vi "Gr_resistance_lockin_using_Rbox_probe.vi"() -> ()   [LabVIEW 2024]
uses:
  <vilib>/Analysis/1siggen.llb/Ramp Pattern by Delta.vi
  <vilib>/Utility/file.llb/Write Delimited Spreadsheet (DBL).vi
  <vilib>/Utility/file.llb/Write Delimited Spreadsheet (string).vi
  <vilib>/Analysis/NI_AALBase.lvlib
  <vilib>/Analysis/NI_AALPro.lvlib
  C:/Users/Public/OneDrive/Desktop/Keithley_2450_2470_1_4_0_LV2015_NewReadme2_2450-LV2015-1.4.0/Keithley 2450/Keithley 2450.lvlib
panel:
  out "Rgr vs Vb":cluster{dbl[], dbl[]}(graph)
  in  "Measurement Count":u32=10
  in  "reset?":bool
  in  "save data":string="H:\\My Drive\\Lab\\PPMS\\Measurement\\GaN_1000C_2min_34_56"
  in  "lockin_avgs":i32=10
  out "std voltage measured":dbl format="%0.2f"
  out "mean voltage measured":dbl=6.7979141 format="%0.4f"
  out "std current measured":dbl=1.0038305493714546e-08 format="%0.5e"
  out "mean current measured":dbl=1.7421272433999997e-09 format="%.4e"
  in  "VISA resource name 2450":refnum<visa-resource-name>="GPIB0::1::INSTR"
  in  "Current Limit":dbl=5e-08
  out "Vb":dbl
  in  "loop?":bool=TRUE
  in  "Vb end (V)":dbl format="%#.4f"
  in  "Vb step (mV)":dbl format="%#_4f"
  in  "Vb start (V)":dbl format="%#.4f"
  out "R_gr":dbl
  out "slope":dbl format="%#_14f"
  out "Vdev":dbl format="%#_14f"
  in  "lockinwait":u32=50
  out "Vbox":dbl format="%#_14f"
  out "Vref vs Idev":cluster{dbl[], dbl[]}[](graph)
  out "Ibox":dbl format="%#_14f"
  in  "Rbox":dbl format="%#_20f"
  out "Sin voltage in":dbl=1.0 format="%#_13f"
  in  "Vmax":dbl format="%.3f"
  in  "Vstep":dbl format="%.5f"
  in  "Vmin":dbl format="%.3f"
  in  "A frequency":dbl=26.7 format="%#_13g"
  in  "B input Connection":u16(ring)=1 items=["Single-Ended Voltage", "Differential Voltage", "1 MOhm Current Gain", "100 MOhm Current Gain"]
  in  "B Reference Source":u8(ring)=1 items=["External", "Internal", "Internal Sweep"]
  in  "B Sensitivity":u16(ring)=26 items=["1 nV/fA", "2 nV/fA", "5 nV/fA", "10 nV/fA", "20 nV/fA", "50 nV/fA", "100 nV/fA", "200 nV/fA", "500 nV/fA", "1 uV/pA", "2 uV/pA", "5 uV/pA", "10 uV/pA", "20 uV/pA", "50 uV/pA", "100 uV/pA", "200 uV/pA", "500 uV/pA", "1 mV/nA", "2 mV/nA", "5 mV/nA", "10 mV/nA", "20 mV/nA", "50 mV/nA", "100 mV/nA", "200 mV/nA", "500 mV/nA", "1 V/uA"]
  in  "LOCKIN1 address":refnum<visa-resource-name>="COM3"
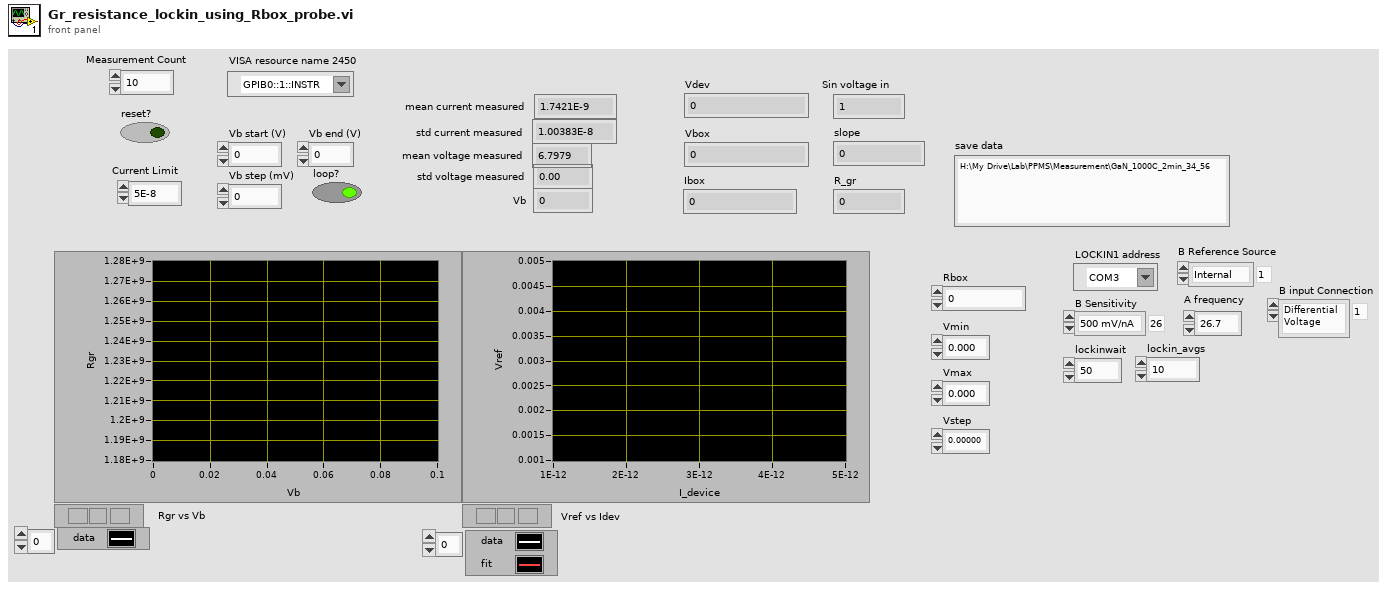
[diagram p1: front panel]
types:
  T1 = enum16{"open", "replace", "create", "open or create", "replace or create", "replace or create with confirmation"}
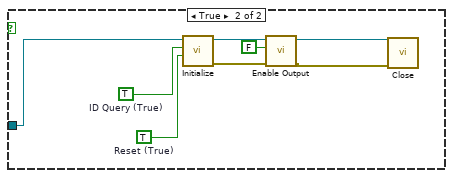
[diagram p3: hidden frame]
diagram:
  w2 = 0
  n1 = Initialize Array(w2, w2) -> (w1:i32[])
  n2 = case shown="False" "reset?" {
    tunnel: "VISA resource name 2450" -> [w10 w581]
    tunnel: w1 -> [w9 _]
    frame False {
      w7 = 0
      w8 = 0
      w17 = TRUE
      n3 = Negate(x="Vb step (mV)") -> (-x=w28:dbl)
      n4 = call-poly <vilib>:"Ramp Pattern.vi"("start"="Vb start (V)", "end"="Vb end (V)", "delta"="Vb step (mV)") -> ("samples"=w24:i32, "Ramp Pattern"=w26:dbl[])  [unwired: 6 in, 1 out]
      n5 = call-poly <vilib>:"Ramp Pattern.vi"("start"="Vb end (V)", "end"="Vb start (V)", "delta"=w28) -> ("samples"=w23:i32, "Ramp Pattern"=w25:dbl[])  [unwired: 6 in, 1 out]
      n6 = case shown="True" "loop?" {
        tunnel: w26 -> [w31 w38]
        tunnel: w25 -> [_ w37]
        tunnel: [w31 w33] -> w20
        tunnel: w24 -> [w32 w35]
        tunnel: [w32 w34] -> w21
        tunnel: w23 -> [_ w36]
        frame False {
        }
        frame True {
          n7 = Add(x=w35, y=w36) -> (x+y=w34:i32)
          n8 = Build Array (concatenate)(w38, w37) -> (w33:dbl[])
        }
      }
      n9 = Concatenate Strings("save data", ".txt" ("string")) -> (w12:string)
      n10 = String To Path(string=w12) -> (path=w19:path)
      n11 = call-poly <vilib>:"Write Delimited Spreadsheet.vi"("file path (dialog if empty)"=w19, "append to file? (new file:F)"=w17) -> ("new file path (Not A Path if cancelled)"=w18:path)  [unwired: 12 in, 1 out]
      n12 = Build Array("# Vb_set(V) Vb_meas(V) R_Gr(Ohm) Ib(uA) " ("string")) -> (w15:string[])
      n13 = Initialize Array(w7, w7) -> (w6:i32[])
      n14 = Initialize Array(w8, w8) -> (w5:i32[])
      n15 = call-poly <vilib>:"Write Delimited Spreadsheet.vi"("file path (dialog if empty)"=w18, "1D data"=w15, "append to file? (new file:F)"=w17) -> ("new file path (Not A Path if cancelled)"=w14:path)  [unwired: 11 in, 1 out]
      n16 = for {
        N: w21 -> [_]
        tunnel: w20 -> [w71] mode=indexing
        tunnel: w10 -> [w99]
        tunnel: w14 -> [w98]
        tunnel: "save data" -> [w81]
        shift-right: [w62] -> _
        shift-left: w9 -> [w72]
        shift-right: [w40] -> _
        shift-left: w6 -> [w59]
        shift-right: [w43] -> _
        shift-left: w5 -> [w52]
        i -> [w39]
        n17 = flat-sequence {
          tunnel: w71 -> [w142]
          tunnel: [w142] -> w100
          tunnel: w99 -> [w154]
          tunnel: [w153] -> w88
          tunnel: [w152] -> w82
          tunnel: w72 -> [w143]
          tunnel: w71 -> [_]
          tunnel: [w143] -> w68
          tunnel: [w140] -> w60
          tunnel: w59 -> [w139]
          tunnel: [w139] -> w58
          tunnel: w52 -> [w138]
          tunnel: [w138] -> w46
          tunnel: [w262] -> w131
          tunnel: [w261] -> w130
          tunnel: ["Rbox"] -> w102
          tunnel: [w257] -> w129
          tunnel: ["Rbox"] -> w128
          tunnel: [w248] -> w127
          tunnel: w100 -> [w248]
          tunnel: [w254] -> w89
          tunnel: w88 -> [w254]
          tunnel: [w253] -> w83
          tunnel: w82 -> [w253]
          tunnel: w81 -> [w252]
          tunnel: ["A frequency"] -> w79
          tunnel: [w250] -> w73
          tunnel: [w249] -> w69
          tunnel: w68 -> [w249]
          tunnel: w60 -> [_]
          tunnel: w58 -> [w244]
          tunnel: [w244] -> w57
          tunnel: [w243] -> w47
          tunnel: w46 -> [w243]
          tunnel: w39 -> [w240]
          tunnel: w131 -> [w296]
          tunnel: [w296] -> w126
          tunnel: w130 -> [w295]
          tunnel: [w295] -> w125
          tunnel: [w279] -> w124
          tunnel: w129 -> [w294]
          tunnel: w128 -> [w291]
          tunnel: ["lockinwait"] -> w101
          tunnel: w127 -> [w273]
          tunnel: [w273] -> w94
          tunnel: [w272] -> w90
          tunnel: w89 -> [w272]
          tunnel: [w271] -> w84
          tunnel: w83 -> [w271]
          tunnel: [w269] -> w80
          tunnel: w79 -> [w269]
          tunnel: [w267] -> w74
          tunnel: w73 -> [w267]
          tunnel: [w266] -> w70
          tunnel: w69 -> [w266]
          tunnel: w57 -> [w265]
          tunnel: [w265] -> w56
          tunnel: [w264] -> w48
          tunnel: w47 -> [w264]
          tunnel: [w320] -> w123
          tunnel: [w314] -> w122
          tunnel: w126 -> [w312]
          tunnel: w125 -> [w313]
          tunnel: [w311] -> w121
          tunnel: w124 -> [w311]
          tunnel: [w304] -> w95
          tunnel: w94 -> [w304]
          tunnel: [w303] -> w91
          tunnel: w90 -> [w303]
          tunnel: [w302] -> w85
          tunnel: w84 -> [w302]
          tunnel: w80 -> [w301]
          tunnel: [w300] -> w75
          tunnel: w74 -> [w300]
          tunnel: w70 -> [w299]
          tunnel: [w299] -> w66
          tunnel: w56 -> [w298]
          tunnel: [w298] -> w55
          tunnel: [w297] -> w49
          tunnel: w48 -> [w297]
          tunnel: w123 -> [w331]
          tunnel: w122 -> [w332]
          tunnel: [w332] -> w120
          tunnel: [w331] -> w119
          tunnel: [w330] -> w118
          tunnel: w121 -> [w330]
          tunnel: [w328] -> w96
          tunnel: w95 -> [w328]
          tunnel: [w327] -> w92
          tunnel: w91 -> [w327]
          tunnel: [w326] -> w86
          tunnel: w85 -> [w326]
          tunnel: [w325] -> w76
          tunnel: w75 -> [w325]
          tunnel: [w324] -> w67
          tunnel: w66 -> [w324]
          tunnel: w55 -> [w323]
          tunnel: [w323] -> w54
          tunnel: [w322] -> w50
          tunnel: w49 -> [w322]
          tunnel: w104 -> [w357]
          tunnel: w103 -> [w356]
          tunnel: w120 -> [w355]
          tunnel: w119 -> [w354]
          tunnel: w118 -> [w353]
          tunnel: [w346] -> w117
          tunnel: [w345] -> w116
          tunnel: [w344] -> w115
          tunnel: [w343] -> w114
          tunnel: [w343] -> w113
          tunnel: [w342] -> w112
          tunnel: w102 -> [w341]
          tunnel: w101 -> [w340]
          tunnel: [w339] -> w97
          tunnel: w96 -> [w339]
          tunnel: [w338] -> w93
          tunnel: w92 -> [w338]
          tunnel: [w337] -> w87
          tunnel: w86 -> [w337]
          tunnel: [w336] -> w77
          tunnel: w76 -> [w336]
          tunnel: w67 -> [w335]
          tunnel: [w335] -> w64
          tunnel: w54 -> [w334]
          tunnel: [w334] -> w53
          tunnel: [w333] -> w51
          tunnel: w50 -> [w333]
          tunnel: w117 -> [w543]
          tunnel: w116 -> [w544]
          tunnel: w115 -> [w549]
          tunnel: w114 -> [w550]
          tunnel: w113 -> [w551]
          tunnel: w112 -> [w555]
          tunnel: [w541] -> w111
          tunnel: [w540] -> w110
          tunnel: w98 -> [w539]
          tunnel: w97 -> [w528]
          tunnel: w93 -> [w538]
          tunnel: w87 -> [w537]
          tunnel: [w534] -> w78
          tunnel: w77 -> [w534]
          tunnel: [w532] -> w65
          tunnel: w64 -> [w532]
          tunnel: [w528] -> w61
          tunnel: w53 -> [w530]
          tunnel: w51 -> [w529]
          tunnel: [w527] -> w44
          tunnel: [w526] -> w41
          tunnel: [w574] -> w109
          tunnel: w111 -> [w574]
          tunnel: [w573] -> w108
          tunnel: w110 -> [w573]
          tunnel: w78 -> [w570]
          tunnel: w65 -> [w564]
          tunnel: [w562] -> w63
          tunnel: w61 -> [w563]
          tunnel: [w560] -> w45
          tunnel: w44 -> [w560]
          tunnel: [w559] -> w42
          tunnel: w41 -> [w559]
          tunnel: w109 -> [w580]
          tunnel: w108 -> [w579]
          tunnel: [w578] -> w62
          tunnel: w63 -> [w578]
          tunnel: [w577] -> w43
          tunnel: w45 -> [w577]
          tunnel: [w576] -> w40
          tunnel: w42 -> [w576]
          frame #0 {
            n18 = flat-sequence {
              tunnel: w154 -> [w170]
              tunnel: w142 -> [w155]
              tunnel: [w164] -> w137
              tunnel: [w163] -> w135
              tunnel: ["Measurement Count"] -> w133
              tunnel: w137 -> [w192]
              tunnel: [w192] -> w136
              tunnel: w135 -> [w191]
              tunnel: [w191] -> w134
              tunnel: w133 -> [w190]
              tunnel: [w190] -> w132
              tunnel: [w194] -> w151
              tunnel: w136 -> [w199]
              tunnel: w134 -> [w198]
              tunnel: [w197] -> w150
              tunnel: [w196] -> w149
              tunnel: w132 -> [w193]
              tunnel: [w193] -> w144
              tunnel: [w214] -> w148
              tunnel: w151 -> [w213]
              tunnel: [w213] -> w147
              tunnel: w150 -> [w219]
              tunnel: w149 -> [w218]
              tunnel: [w217] -> w146
              tunnel: [w216] -> w145
              tunnel: w144 -> [w211]
              tunnel: [w232] -> w153
              tunnel: w148 -> [w232]
              tunnel: [w231] -> w152
              tunnel: w147 -> [w231]
              tunnel: w146 -> [w234]
              tunnel: w145 -> [w235]
              frame #0 {
                w172 = u16 2 items=["Volts", "Current", "Resistance"] ("Function (0: Volts)")
                w179 = u16 0 items=["Voltage", "Current"]  # Source Mode  (0: Voltage)
                w180 = u16 1 items=["Volts", "Current", "Auto Resistance", "Manual Resistance", "Digitize Voltage", "Digitize Current"]  # Measurement Mode
                w171 = TRUE  # Enable Auto Range (T:Enable)
                w181 = u16 1 items=["Volts", "Current", "Resistance"]  # Function (0: Volts)
                w182 = u16 0 items=["Volts", "Current", "Resistance"]  # Function (0: Volts)
                w177 = FALSE  # Reset (True)
                n19 = call "Initialize.vi"("Reset (True)"=w177, "VISA resource name"=w170) -> ("error out"=w156:errorcluster, "VISA resource name out"=w161:refnum<visa-resource-name>)  [unwired: 8 in]
                n20 = call "Clear Buffer.vi"("VISA resource name"=w161, "error in (no error)"=w156) -> ("VISA resource name out"=w160:refnum<visa-resource-name>, "error out"=w157:errorcluster)  [unwired: 12 in]
                n21 = call "Clear Buffer Statistics.vi"("VISA resource name"=w160, "error in (no error)"=w157) -> ("VISA resource name out"=w159:refnum<visa-resource-name>, "error out"=w158:errorcluster)  [unwired: 12 in]
                n22 = call "Configure Measurement Range.vi"("error in (no error)"=w158, "Enable Auto Range (T:Enable)"=w171, "Function (0: Volts)"=w182, "VISA resource name"=w159) -> ("error out"=w184:errorcluster, "VISA resource name out"=w183:refnum<visa-resource-name>)  [unwired: 6 in]
                n23 = call "Configure Measurement Range.vi"("error in (no error)"=w184, "Enable Auto Range (T:Enable)"=w171, "Function (0: Volts)"=w181, "VISA resource name"=w183) -> ("error out"=w175:errorcluster, "VISA resource name out"=w176:refnum<visa-resource-name>)  [unwired: 6 in]
                n24 = call "Configure Measurement Range.vi"("error in (no error)"=w175, "Enable Auto Range (T:Enable)"=w171, "Function (0: Volts)"=w172, "VISA resource name"=w176) -> ("error out"=w174:errorcluster, "VISA resource name out"=w173:refnum<visa-resource-name>)  [unwired: 6 in]
                n25 = call "Configure Output.vi"("VISA resource name"=w173, "Source Level (0)"=w155, "Source Mode  (0: Voltage)"=w179, "Source Limit Level (0.1)"="Current Limit", "error in (no error)"=w174) -> ("VISA resource name out"=w185:refnum<visa-resource-name>, "error out"=w186:errorcluster)  [unwired: 9 in]
                n26 = call "Configure Source Function.vi"("error in (no error)"=w186, "Function (0: Volts)"=w179, "VISA resource name"=w185) -> ("error out"=w187:errorcluster, "VISA resource name out"=w188:refnum<visa-resource-name>)  [unwired: 7 in]
                n27 = call "Configure Measurement Function.vi"("error in (no error)"=w187, "Function (0: Volts)"=w180, "VISA resource name"=w188) -> ("error out"=w168:errorcluster, "VISA resource name out"=w169:refnum<visa-resource-name>)  [unwired: 7 in]
                n28 = call "Set Measurement Count.vi"("error in (no error)"=w168, "Measurement Count"="Measurement Count", "VISA resource name"=w169) -> ("error out"=w166:errorcluster, "VISA resource name out"=w167:refnum<visa-resource-name>)  [unwired: 7 in]
                n29 = call "Enable Output.vi"("error in (no error)"=w166, "Enable Output (T: Enable)"=TRUE, "VISA resource name"=w167) -> ("error out"=w163:errorcluster, "VISA resource name out"=w164:refnum<visa-resource-name>)  [unwired: 7 in]
              }
              frame #1 {
                n30 = Wait (ms)(milliseconds to wait=200) -> ()  [unwired: 1 out]
              }
              frame #2 {
                w200 = 1000000.0 ("Timeout (10000 ms)")
                n31 = call "Make Reading and Store in Buffer.vi"("VISA resource name"=w199, "error in (no error)"=w198) -> ("VISA resource name out"=w208:refnum<visa-resource-name>, "error out"=w209:errorcluster)  [unwired: 12 in]
                n32 = call "Read (Multiple Points).vi"("VISA resource name"=w208, "Start Index (1)"=u32 1, "End Index (1)"=w193, "error in (no error)"=w209) -> ("VISA resource name out"=w197:refnum<visa-resource-name>, "Data out"=w203:string, "error out"=w196:errorcluster)  [unwired: 9 in]
                n33 = Spreadsheet String To Array(delimiter (Tab)=",", format string="%s", spreadsheet string=w203, array type (2D Dbl)=dbl[] []) -> (array=w202:dbl[])
                n34 = call <vilib>:"Std Deviation and Variance.vi"("X"=w202) -> ("mean"=w195:dbl, "standard deviation"=w201:dbl)  [unwired: 1 in, 1 out]
                "mean current measured" <- w195
                "std current measured" <- w201
                n35 = Multiply(x=w201, y=w200) -> ()  [unwired: 1 out]
                n36 = Multiply(x=w200, y=w195) -> (x*y=w194:dbl)
              }
              frame #3 {
                n37 = call "Configure Measurement Function.vi"("error in (no error)"=w218, "VISA resource name"=w219) -> ("error out"=w226:errorcluster, "VISA resource name out"=w230:refnum<visa-resource-name>)  [unwired: 8 in]
                n38 = call "Set Measurement Count.vi"("error in (no error)"=w226, "Measurement Count"=w211, "VISA resource name"=w230) -> ("error out"=w227:errorcluster, "VISA resource name out"=w225:refnum<visa-resource-name>)  [unwired: 7 in]
                n39 = Increment(x=w211) -> (x+1=w212:u32)
                n40 = Add(x=w211, y=w211) -> (x+y=w210:u32)
                n41 = call "Make Reading and Store in Buffer.vi"("VISA resource name"=w225, "error in (no error)"=w227) -> ("VISA resource name out"=w229:refnum<visa-resource-name>, "error out"=w228:errorcluster)  [unwired: 12 in]
                n42 = call "Read (Multiple Points).vi"("VISA resource name"=w229, "Start Index (1)"=w212, "End Index (1)"=w210, "error in (no error)"=w228) -> ("VISA resource name out"=w216:refnum<visa-resource-name>, "Data out"=w221:string, "error out"=w217:errorcluster)  [unwired: 9 in]
                n43 = Spreadsheet String To Array(delimiter (Tab)=",", format string="%s", spreadsheet string=w221, array type (2D Dbl)=dbl[] []) -> (array=w220:dbl[])
                n44 = call <vilib>:"Std Deviation and Variance.vi"("X"=w220) -> ("mean"=w214:dbl, "standard deviation"=→"std voltage measured":dbl)  [unwired: 1 in, 1 out]
                "mean voltage measured" <- w214
              }
              frame #4 {
                n45 = call "Enable Output.vi"("error in (no error)"=w234, "Enable Output (T: Enable)"=TRUE, "VISA resource name"=w235) -> ("error out"=w237:errorcluster, "VISA resource name out"=w238:refnum<visa-resource-name>)  [unwired: 7 in]
                n46 = call "Close.vi"("error in (no error)"=w237, "VISA resource name"=w238) -> ("error out"=w236:errorcluster)  [unwired: 9 in]
                n47 = call <vilib>:"Simple Error Handler.vi"("error in (no error)"=w236) -> ()  [unwired: 4 in, 5 out]
              }
            }
            n48 = Search 1D Array(1D array=w143, element=w142) -> (index of element=w141:i32)  [unwired: 1 in]
            n49 = Less Than 0?(x=w141) -> (x < 0?=w140:bool)
          }
          frame #1 {
            n50 = Multiply(x=w248, y=1000.0) -> (x*y=w247:dbl)
            n51 = Round To Nearest(number=w247) -> (nearest integer value=w246:dbl)
            n52 = Format Into String(format string="%d", w246) -> (resulting string=w259:string)  [unwired: 2 in, 1 out]
            n53 = Format Into String(w240) -> (resulting string=w239:string)  [unwired: 3 in, 1 out]
            n54 = Concatenate Strings(w252, "_VI_data_Vb" ("string"), w259, "mV__" ("string"), w239, "__.txt" ("string")) -> (w250:string)
            n55 = local read "LOCKIN1 address"() -> (w263:refnum<visa-resource-name>)
            n56 = String To Path(string=w250) -> (path=w257:path)
            n57 = Open/Create/Replace File(file path (use dialog)=w257, operation (0:open)=T1."open or create") -> ()  [unwired: 4 in, 3 out]
            n58 = call "OE1022D_OpenDevice.vi"("VISA resource name"=w263) -> ("VISA资源名称输出"=w262:refnum<visa-resource-name>, "错误输出"=w261:errorcluster)  [unwired: 17 in]
          }
          frame #2 {
            w277 = TRUE
            n59 = Format Into String(initial string="# Rbox (Ohm) = ", w291) -> (resulting string=w293:string)  [unwired: 2 in, 1 out]
            n60 = Format Into String(initial string="# Freq (Hz) = ", w269) -> (resulting string=w268:string)  [unwired: 2 in, 1 out]
            n61 = Build Array(w293) -> (w290:string[])
            n62 = Format Into String(initial string="# Vb(V) = ", w273) -> (resulting string=w278:string)  [unwired: 2 in, 1 out]
            n63 = Format Into String(initial string="# Lockin wait time (ms) = ", "lockinwait") -> (resulting string=w285:string)  [unwired: 2 in, 1 out]
            n64 = Build Array(w278) -> (w274:string[])
            n65 = call-poly <vilib>:"Write Delimited Spreadsheet.vi"("file path (dialog if empty)"=w294, "1D data"=w290, "append to file? (new file:F)"=w277) -> ("new file path (Not A Path if cancelled)"=w289:path)  [unwired: 11 in, 1 out]
            n66 = Build Array(w285) -> (w284:string[])
            n67 = Build Array(w268) -> (w281:string[])
            n68 = Build Array("# Vref(V) Vbox(V) Ibox(uA) Rdev(Ohm) theta(deg)" ("format string")) -> (w275:string[])
            n69 = call-poly <vilib>:"Write Delimited Spreadsheet.vi"("file path (dialog if empty)"=w289, "1D data"=w284, "append to file? (new file:F)"=w277) -> ("new file path (Not A Path if cancelled)"=w287:path)  [unwired: 11 in, 1 out]
            n70 = call-poly <vilib>:"Write Delimited Spreadsheet.vi"("file path (dialog if empty)"=w287, "1D data"=w281, "append to file? (new file:F)"=w277) -> ("new file path (Not A Path if cancelled)"=w282:path)  [unwired: 11 in, 1 out]
            n71 = call-poly <vilib>:"Write Delimited Spreadsheet.vi"("file path (dialog if empty)"=w282, "1D data"=w274, "append to file? (new file:F)"=w277) -> ("new file path (Not A Path if cancelled)"=w280:path)  [unwired: 11 in, 1 out]
            n72 = call-poly <vilib>:"Write Delimited Spreadsheet.vi"("file path (dialog if empty)"=w280, "1D data"=w275, "append to file? (new file:F)"=w277) -> ("new file path (Not A Path if cancelled)"=w279:path)  [unwired: 11 in, 1 out]
          }
          frame #3 {
            w316 = u8 1 items=["Channel A", "Channel B"] ("OE1022D A/B")
            n73 = call "OE1022D_Configure Reference Source.vi"("VISA resource name"=w312, "OE1022D A/B"=w316, "Reference Source"="B Reference Source", "error in (no error)"=w313) -> ("VISA resource name out"=w310:refnum<visa-resource-name>, "error out"=w309:errorcluster)  [unwired: 14 in]
            n74 = call "OE1022D_Configure Frequency.vi"("VISA resource name"=w310, "OE1022D A/B"=w316, "Internal Frequency(Hz)"=w301, "error in (no error)"=w309) -> ("VISA resource name out"=w319:refnum<visa-resource-name>, "error out"=w318:errorcluster)  [unwired: 14 in]
            n75 = call "OE1022D_Configure Ref Phase Channel A.vi"("VISA resource name"=w319, "Reference Source"="B Reference Source", "Internal Frequency(Hz)"=w301, "error in (no error)"=w318) -> ("VISA resource name out"=w305:refnum<visa-resource-name>, "error out"=w306:errorcluster)  [unwired: 14 in]
            n76 = call "OE1022D_Configure Sensitivity.vi"("VISA resource name"=w305, "OE1022D A/B"=w316, "Sensitivity"="B Sensitivity", "error in (no error)"=w306) -> ("VISA resource name out"=w307:refnum<visa-resource-name>, "error out"=w308:errorcluster)  [unwired: 14 in]
            n77 = call "OE1022D_Configure Input Filter.vi"("VISA resource name"=w307, "Input Source"="B input Connection", "OE1022D A/B"=w316, "error in (no error)"=w308) -> ("VISA resource name out"=w314:refnum<visa-resource-name>, "error out"=w320:errorcluster)  [unwired: 10 in]
          }
          frame #4 {
            n78 = Wait (ms)(milliseconds to wait=500) -> ()  [unwired: 1 out]
          }
          frame #5 {
            w348 = 0
            w350 = 0
            w352 = 0
            n79 = Initialize Array(w352, w352) -> (w351:i32[])
            n80 = Initialize Array(w350, w350) -> (w349:i32[])
            n81 = Initialize Array(w348, w348) -> (w347:i32[])
            n82 = for {
              N: w357 -> [_]
              tunnel: w356 -> [w425] mode=indexing
              tunnel: w355 -> [w427]
              tunnel: w354 -> [w426]
              tunnel: w353 -> [w424]
              shift-right: [w406] -> _
              shift-left: w351 -> [w411]
              shift-right: [w400] -> w344
              shift-left: w349 -> [w405]
              shift-right: [w391] -> w343
              shift-left: w347 -> [w397]
              tunnel: [w361] -> w345
              tunnel: [w358] -> w346
              tunnel: [w365] -> w342
              tunnel: w341 -> [w364]
              tunnel: w340 -> [w363]
              n83 = flat-sequence {
                tunnel: w427 -> [w436]
                tunnel: w426 -> [w435]
                tunnel: w425 -> [w428]
                tunnel: [w434] -> w390
                tunnel: [w433] -> w388
                tunnel: [w428] -> w386
                tunnel: [w432] -> w384
                tunnel: w411 -> [w432]
                tunnel: [w431] -> w382
                tunnel: w405 -> [w431]
                tunnel: w397 -> [w430]
                tunnel: [w429] -> w380
                tunnel: [w428] -> w367
                tunnel: w390 -> [w448]
                tunnel: [w448] -> w389
                tunnel: w388 -> [w447]
                tunnel: [w447] -> w387
                tunnel: w386 -> [w446]
                tunnel: [w446] -> w385
                tunnel: w384 -> [w445]
                tunnel: [w445] -> w383
                tunnel: w382 -> [w444]
                tunnel: [w444] -> w381
                tunnel: w380 -> [w443]
                tunnel: [w443] -> w379
                tunnel: w367 -> [w442]
                tunnel: [w442] -> w366
                tunnel: w363 -> [w441]
                tunnel: w389 -> [w460]
                tunnel: w387 -> [w459]
                tunnel: [w458] -> w422
                tunnel: [w457] -> w421
                tunnel: w385 -> [w465]
                tunnel: [w465] -> w416
                tunnel: [w454] -> w412
                tunnel: w383 -> [w464]
                tunnel: [w463] -> w407
                tunnel: w381 -> [w462]
                tunnel: [w462] -> w403
                tunnel: w379 -> [w461]
                tunnel: [w461] -> w393
                tunnel: [w454] -> w375
                tunnel: [w455] -> w371
                tunnel: w366 -> [w453]
                tunnel: [w474] -> w423
                tunnel: w422 -> [w474]
                tunnel: w421 -> [w473]
                tunnel: [w473] -> w420
                tunnel: [w472] -> w417
                tunnel: w416 -> [w472]
                tunnel: [w471] -> w413
                tunnel: w412 -> [w471]
                tunnel: [w470] -> w408
                tunnel: w407 -> [w470]
                tunnel: [w469] -> w404
                tunnel: w403 -> [w469]
                tunnel: [w468] -> w394
                tunnel: w393 -> [w468]
                tunnel: [w467] -> w376
                tunnel: w375 -> [w467]
                tunnel: w371 -> [w466]
                tunnel: [w466] -> w370
                tunnel: w423 -> [w482]
                tunnel: w420 -> [w479]
                tunnel: [w488] -> w418
                tunnel: w417 -> [w488]
                tunnel: [w487] -> w414
                tunnel: w413 -> [w487]
                tunnel: [w486] -> w409
                tunnel: w408 -> [w486]
                tunnel: w404 -> [w485]
                tunnel: [w485] -> w401
                tunnel: [w484] -> w395
                tunnel: w394 -> [w484]
                tunnel: [w483] -> w377
                tunnel: w376 -> [w483]
                tunnel: [w480] -> w374
                tunnel: [w481] -> w373
                tunnel: w370 -> [w478]
                tunnel: [w476] -> w369
                tunnel: [w497] -> w419
                tunnel: w418 -> [w497]
                tunnel: [w496] -> w415
                tunnel: w414 -> [w496]
                tunnel: [w495] -> w410
                tunnel: w409 -> [w495]
                tunnel: [w494] -> w402
                tunnel: w401 -> [w494]
                tunnel: [w493] -> w396
                tunnel: w395 -> [w493]
                tunnel: [w492] -> w378
                tunnel: w377 -> [w492]
                tunnel: w374 -> [w491]
                tunnel: w373 -> [w489]
                tunnel: [w491] -> w372
                tunnel: [w489] -> _
                tunnel: w369 -> [w490]
                tunnel: [w490] -> w368
                tunnel: [w489] -> w359
                tunnel: w424 -> [w516]
                tunnel: w419 -> [w512]
                tunnel: w415 -> [w511]
                tunnel: w410 -> [w509]
                tunnel: w402 -> [w508]
                tunnel: [w509] -> w399
                tunnel: [w507] -> w398
                tunnel: w396 -> [w506]
                tunnel: [w506] -> w392
                tunnel: w378 -> [w505]
                tunnel: w372 -> [w503]
                tunnel: w368 -> [_]
                tunnel: [w504] -> w365
                tunnel: w364 -> [w504]
                tunnel: [w503] -> w362
                tunnel: [w502] -> w360
                tunnel: w359 -> [w502]
                tunnel: [w518] -> w400
                tunnel: [w525] -> w406
                tunnel: w399 -> [w525]
                tunnel: w398 -> [w518]
                tunnel: [w519] -> w391
                tunnel: w392 -> [w519]
                tunnel: [w524] -> w361
                tunnel: w362 -> [w524]
                tunnel: [w523] -> w358
                tunnel: w360 -> [w523]
                frame #0 {
                  n84 = Build Array (concatenate)(w430, w428) -> (w429:dbl[])
                  n85 = Format Into String(format string="SLVLD2,%.4f;", w428) -> (resulting string=w439:string)  [unwired: 2 in, 1 out]
                  n86 = Concatenate Strings(w439, "\r") -> (w440:string)
                  n87 = VISA Write(VISA resource name=w436, write buffer=w440, error in (no error)=w435) -> (VISA resource name out=w434:refnum<visa-resource-name>, error out=w433:errorcluster)  [unwired: 1 out]
                  "Sin voltage in" <- w428
                }
                frame #1 {
                  n88 = Wait (ms)(milliseconds to wait=w441) -> ()  [unwired: 1 out]
                }
                frame #2 {
                  w456 = u16 2 items=["X", "Y", "R", "Theta", "Frequency", "Noise", "Xh1", "Yh1", "Rh1", "Theta h1", "Xh2", "Yh2", "Rh2", "Theta h2"] ("Parameter 2")
                  w455 = 1
                  n89 = call "OE1022D_Read 1 parameter_mean_and_std.vi"("Num Averages"="lockin_avgs", "Parameter 2"=w456, "错误输入（无错误）"=w459, "Channel (0: A)"=w455, "VISA resource name"=w460) -> ("error out"=w458:errorcluster, "Measurement"=w454:dbl, "VISA resource name out"=w457:refnum<visa-resource-name>)  [unwired: 3 in, 1 out]
                  "Vbox" <- w454
                  n90 = Subtract(x=w453, y=w454) -> (x-y=w452:dbl)
                  n91 = Build Array (concatenate)(w464, w454) -> (w463:dbl[])
                  n92 = Multiply(x=w452, y=1000000.0) -> (x*y=→"Vdev":dbl)
                }
                frame #3 {
                  n93 = Wait (ms)(milliseconds to wait=u32 50) -> ()  [unwired: 1 out]
                }
                frame #4 {
                  w477 = u16 3 items=["X", "Y", "R", "Theta", "Frequency", "Noise", "Xh1", "Yh1", "Rh1", "Theta h1", "Xh2", "Yh2", "Rh2", "Theta h2"] ("Parameter 2")
                  n94 = call "OE1022D_Read 1 parameter_mean_and_std.vi"("Parameter 2"=w477, "错误输入（无错误）"=w482, "Channel (0: A)"=w478, "VISA resource name"=w479) -> ("error out"=w481:errorcluster, "Measurement"=w476:dbl, "VISA resource name out"=w480:refnum<visa-resource-name>)  [unwired: 4 in, 1 out]
                }
                frame #5 {
                  n95 = Wait (ms)(milliseconds to wait=u32 50) -> ()  [unwired: 1 out]
                }
                frame #6 {
                  (unwired) "Vref\nVbox\nIbox\nRdevice\nTheta"
                  n96 = Divide(x=w511, y=w504) -> (x/y=w500:dbl)
                  n97 = Divide(x=w512, y=w500) -> (x/y=w513:dbl)
                  n98 = Build Array (concatenate)(w508, w500) -> (w507:dbl[])
                  n99 = Subtract(x=w513, y=w504) -> (x-y=w510:dbl)
                  n100 = Multiply(x=w500, y=1000000.0) -> (x*y=w499:dbl)
                  "Ibox" <- w499
                  n101 = Build Array(w512, w511, w499, w510, w505) -> (w517:dbl[])
                  n102 = call-poly <vilib>:"Write Delimited Spreadsheet.vi"("file path (dialog if empty)"=w516, "format (%.3f)"="%.12f", "1D data"=w517, "append to file? (new file:F)"=TRUE) -> ()  [unwired: 10 in, 2 out]
                }
                frame #7 {
                  n103 = Bundle(w518, w519) -> (w520:cluster{dbl[], dbl[]})  [unwired: 1 in]
                  n104 = Bundle(w518, w519) -> (w522:cluster{dbl[], dbl[]})  [unwired: 1 in]
                  n105 = Build Array(w522, w520) -> (w521:cluster{dbl[], dbl[]}[])
                  "Vref vs Idev" <- w521
                  n106 = local write "Vref vs Idev"(w521) -> ()
                }
              }
            }
          }
          frame #6 {
            n107 = Bundle(w549, w551) -> (w557:cluster{dbl[], dbl[]})  [unwired: 1 in]
            n108 = call <vilib>:"Linear Fit.vi"("Y"=w549, "X"=w550) -> ("Best Linear Fit"=w554:dbl[], "slope"=w553:dbl)  [unwired: 9 in, 3 out]
            "slope" <- w553
            n109 = Reciprocal(x=w553) -> (1/x=w552:dbl)
            n110 = Bundle("Best Linear Fit"=w554, w551) -> (w556:cluster{"Best Linear Fit":dbl[], dbl[]})  [unwired: 1 in]
            n111 = Format Into String(format string="SLVLD2,%.4f;", 0.001 ("input 1")) -> (resulting string=w547:string)  [unwired: 2 in, 1 out]
            n112 = Subtract(x=w552, y=w555) -> (x-y=w531:dbl)
            "R_gr" <- w531
            n113 = Build Array(w528, w538, w531, w537) -> (w536:dbl[])
            n114 = Build Array(w557, w556) -> (w535:cluster{"Best Linear Fit":dbl[], dbl[]}[])
            n115 = Concatenate Strings(w547, "\r") -> (w548:string)
            n116 = Build Array (concatenate)(w529, w528) -> (w527:dbl[])
            n117 = local write "Vref vs Idev"(w535) -> ()
            n118 = call-poly <vilib>:"Write Delimited Spreadsheet.vi"("file path (dialog if empty)"=w539, "format (%.3f)"="%.12f", "1D data"=w536, "append to file? (new file:F)"=TRUE) -> ()  [unwired: 10 in, 2 out]
            n119 = Build Array (concatenate)(w530, w531) -> (w526:dbl[])
            n120 = VISA Write(VISA resource name=w544, write buffer=w548, error in (no error)=w543) -> (VISA resource name out=w540:refnum<visa-resource-name>, error out=w541:errorcluster)  [unwired: 1 out]
          }
          frame #7 {
            n121 = Concatenate Strings(w570, "_plot" ("format string")) -> (w568:string)
            n122 = String To Path(string=w568) -> (path=w567:path)
            n123 = Bundle(w560, w559) -> (→"Rgr vs Vb":cluster{dbl[], dbl[]})  [unwired: 1 in]
            n124 = Wait (ms)(milliseconds to wait=u32 100) -> ()  [unwired: 1 out]
            n125 = invoke on="Vref vs Idev" class="XYGraph (strict)" method="Export Image"("FileType"=enum32{"BMP", "EPS", "EMF", "PICT"}."BMP" ("File Type"), "Target"=enum32{"File", "Clipboard"}."File", "Path"=w567, "HideGrid"=FALSE ("Hide Grid"), "Overwrite"=TRUE ("Always Overwrite")) -> ()  [unwired: 3 in, 8 out]
            n126 = Build Array (concatenate)(w564, w563) -> (w562:dbl[])
          }
          frame #8 {
            n127 = call "OE1022D_Close.vi"("错误输入（无错误）"=w580, "VISA resource name"=w579) -> ()  [unwired: 1 in, 1 out]
          }
        }
        n128 = call-poly <vilib>:"Ramp Pattern.vi"("start"="Vmin", "end"="Vmax", "delta"="Vstep") -> ("samples"=w104:i32, "Ramp Pattern"=w103:dbl[])  [unwired: 6 in, 1 out]
        "Vb" <- w71
      }
    }
    frame True {
      w587 = TRUE  # Reset (True)
      w588 = TRUE  # ID Query (True)
      n129 = call "Initialize.vi"("Reset (True)"=w587, "ID Query (True)"=w588, "VISA resource name"=w581) -> ("error out"=w586:errorcluster, "VISA resource name out"=w585:refnum<visa-resource-name>)  [unwired: 7 in]
      n130 = call "Enable Output.vi"("error in (no error)"=w586, "Enable Output (T: Enable)"=FALSE, "VISA resource name"=w585) -> ("error out"=w583:errorcluster, "VISA resource name out"=w584:refnum<visa-resource-name>)  [unwired: 7 in]
      n131 = call "Close.vi"("error in (no error)"=w583, "VISA resource name"=w584) -> ()  [unwired: 9 in, 1 out]
    }
  }
